vi "Insert Subsequence.vi"(6 "Insertion Index":i32=-1, 7 "Parent ID":string, 8 "error in (no error)":errorcluster, 9 "Unique ID":string, 10 "Name":string, 11 "Test Executive in":refnum<class "Test Executive.lvclass">) -> (0 "error out":errorcluster, 1 "Replaced?":bool, 3 "Test Executive out":refnum<class "Test Executive.lvclass">, 5 "Unique ID out":string)   [LabVIEW 2017, in "Test Executive.lvlib" / "Test Executive.lvclass"]
uses:
  <vilib>/gpm_packages/@cs/test-executive/Source/Test Executive/TestExecutive/Test Executive.lvclass
  <vilib>/gpm_packages/@cs/test-executive/Source/Test Executive/Subsequence/Subsequence.lvclass
  <vilib>/gpm_packages/@cs/test-executive/Source/Test Executive/TestExecutive/Test Executive.lvclass/Test Executive.ctl
  c37fd379-cacf-4913-81eb-e0a7b8b7285d.vi
  <vilib>/gpm_packages/@cs/linked-list/Source/Linked List/ILinkedList/ILinked List.lvclass
  <vilib>/gpm_packages/@cs/linked-list/Source/Linked List/Linked List Ref/Linked List Ref.lvclass
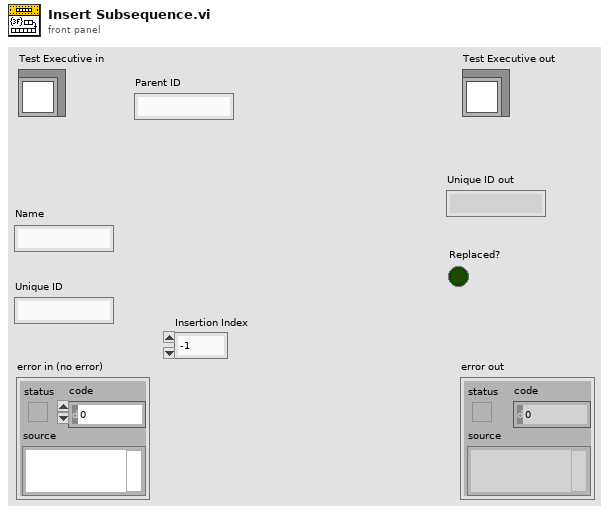
[diagram p1: front panel]
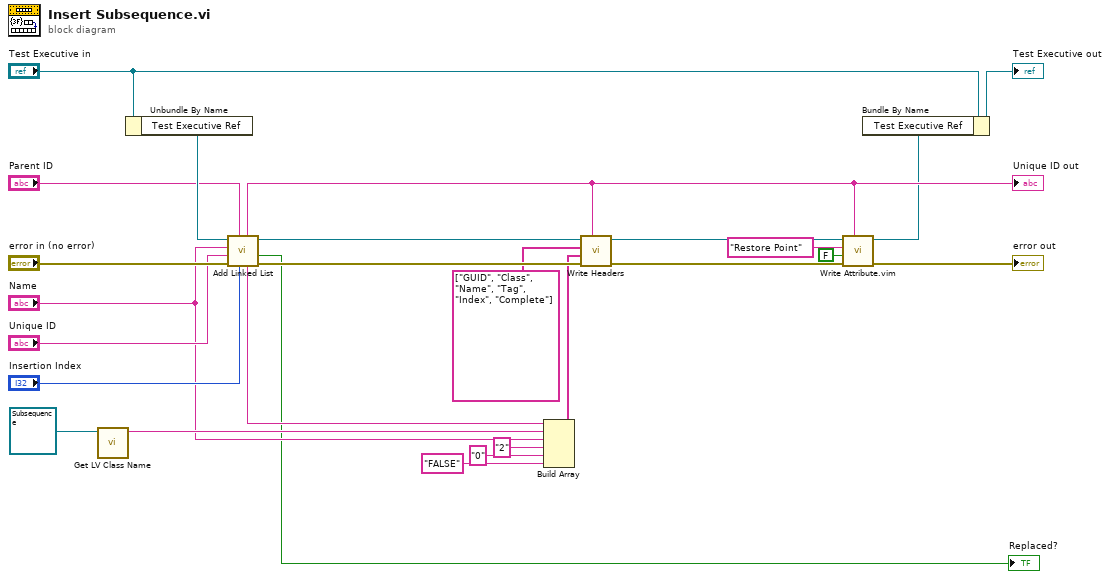
[diagram p0: block diagram]
diagram:
  n1 = call <vilib>:"Get LV Class Name.vi"("object"=refnum<class "Subsequence.lvclass"> refnum ("Test Executive.lvlib:Subsequence.lvclass")) -> ("class name"=w16:string)  [unwired: 9 in, 1 out]
  n2 = Unbundle By Name("Test Executive in") -> ("Test Executive Ref"=w23:refnum<data-value>)
  n3 = call <vilib>:"Add Linked List.vi"("Insertion Index"="Insertion Index", "Parent ID"="Parent ID", "error in (no error)"="error in (no error)", "Linked List ID"="Unique ID", "Name"="Name", "Linked List Ref"=w23) -> ("error out"=w19:errorcluster, "Replaced?"=→"Replaced?":bool, "Linked List Ref out"=w20:refnum<data-value>, "Linked List ID out"=w7:string)  [unwired: 2 in]
  "Unique ID out" <- w7
  n4 = Build Array(w7, w16, "Name", "2" ("element"), "0" ("element"), "FALSE" ("element")) -> (w13:string[])
  n5 = call <vilib>:"Write Headers.vi"("Linked List ID"=w7, "error in (no error)"=w19, "Header Values"=w13, "Header Names"=string[] ["GUID", "Class", "Name", "Tag", "Index", "Complete"], "Linked List Ref"=w20) -> ("error out"=w9:errorcluster, "Linked List Ref out"=w10:refnum<data-value>)  [unwired: 5 in]
  n6 = call "Write Attribute.vim"("Linked List ID"=w7, "error in (no error)"=w9, "Attribute"=FALSE, "Attribute Name"="Restore Point", "Linked List Ref"=w10) -> ("error out"=→"error out":errorcluster, "Linked List Ref out"=w4:refnum<data-value>)  [unwired: 3 in, 2 out]
  n7 = Bundle By Name(cluster="Test Executive in", "Test Executive Ref"=w4) -> (→"Test Executive out":refnum<class "Test Executive.lvclass">)
